vi "[RT] Initialize Simulation.vi"(8 "Error In":errorcluster, 11 "Resource name":T1 caption="RIO Device") -> (0 "Error out":errorcluster, 3 "FPGA VI reference":T2)   [LabVIEW 2017]
uses:
  Controls/eHS FPGA Ref.ctl
  <vilib>/userdefined/High Color/nirio_resource_hc.ctl
  <vilib>/FPGAPlugInAG/cRIO-9039/niLvFpga_Open_cRIO-9039.vi
  <vilib>/rvi/interface/common/dynamic/niFpgaDynamicAddResources.vi
  <vilib>/FPGAPlugInAG/Dynamic/niLvFpga_Download_Dynamic.vi
  <vilib>/FPGAPlugInAG/Dynamic/niLvFpga_Run_Dynamic.vi
  <vilib>/rvi/interface/nirviOpenFPGA/nirviOpenFPGA.xnode
  FPGA Bitfiles/eHS (9039)_Qt9XAGr9Vcg.lvbitx
  <vilib>/rvi/interface/nirviMethod/nirviMethod.xnode
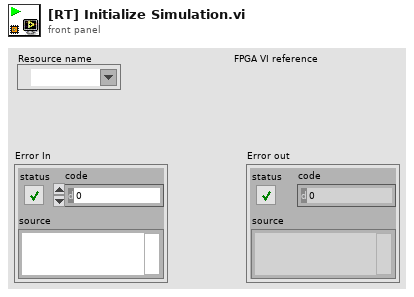
[diagram p1: front panel]
types:
  T1 = typedef "nirio_resource_hc.ctl" = tag
  T2 = typedef "eHS FPGA Ref.ctl" = refnum<k20>
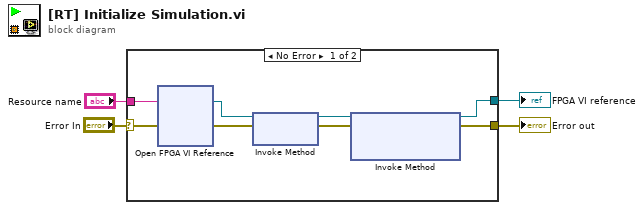
[diagram p0: block diagram]
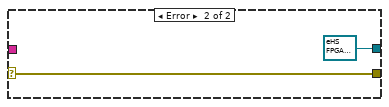
[diagram p2: hidden frame]
diagram:
  n1 = case shown="No Error" "Error In" {
    selector: "Error In" -> [w6 w14]
    tunnel: [w10 w14] -> w4
    tunnel: "Resource name" -> [w9 _]
    tunnel: [w5 T2 refnum ("FPGA VI reference")] -> w1
    frame No Error {
      n2 = xnode "Open FPGA VI Reference"("error in"=w6, "resource name"=w9) -> ("FPGA VI Reference Out"=w12:refnum<k20>, "error out"=w11:errorcluster)
      n3 = xnode "Invoke Method"("FPGA VI Reference In"=w12, "error in"=w11) -> ("FPGA VI Reference Out"=w8:refnum<k20>, "error out"=w7:errorcluster)
      n4 = xnode "Invoke Method"("FPGA VI Reference In"=w8, "error in"=w7) -> ("FPGA VI Reference Out"=w5:refnum<k20>, "error out"=w10:errorcluster)  [unwired: 1 in]
    }
    frame Error {
    }
  }
  "Error out" <- w4
  "FPGA VI reference" <- w1
